vi "Billard2025.vi"(5 "Open PDF":bool=TRUE, 7 "Diamètre balle":i32=13, 8 "ColorchocWin":u32(colorbox), 9 "ColorchocLose":u32(colorbox), 10 "Create scoresheet":bool=TRUE, 11 "Path":path) -> (0 "Error out":errorcluster, 1 "Summary":string)   [LabVIEW 2025]
panel:
  out "?":string="Billard 2025"
  out "BANCKEN Thomas 393134\n\nDELAMARE Romain 373041\n\nDIEBOLD Jules 393356":string="BANCKEN Thomas 393134\n\nDELAMARE Romain 373041\n\nDIEBOLD Jules 393356"
  out "?":string="Auteurs"
  out "PNG Picture":picture
  out "Output cluster":errorcluster
  in  "LineStyle":enum16{"-", "--", ":", "-."}(ring)=enum."--"
  in  "MarkerStyle":enum16{"o", "+", "*", ".", "x", "s", "d"}(ring)=enum."*"
  # "(Doit etre compris entre 10 & 15)"
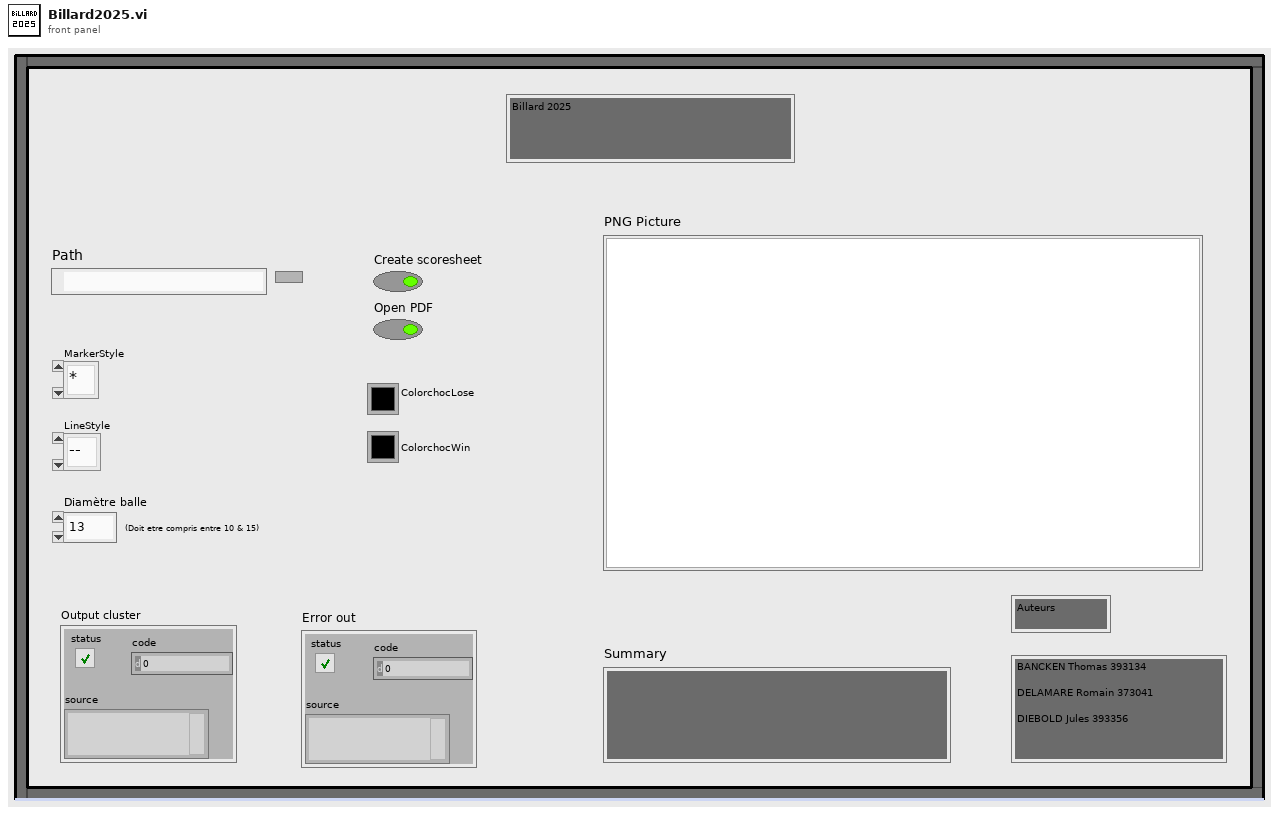
[diagram p1: front panel]
types:
  T1 = cluster{"Bottom":dbl, "Top":dbl, "Left":dbl, "Right":dbl}
  T2 = cluster{"Xr":i32, "Yr":i32, "Sr":i32, "Xy":i32, "Yy":i32, "Sy":i32, "Xw":i32, "Yw":i32, "Sw":i32}
  T3 = enum16{"open", "replace", "create", "open or create", "replace or create", "replace or create with confirmation"}
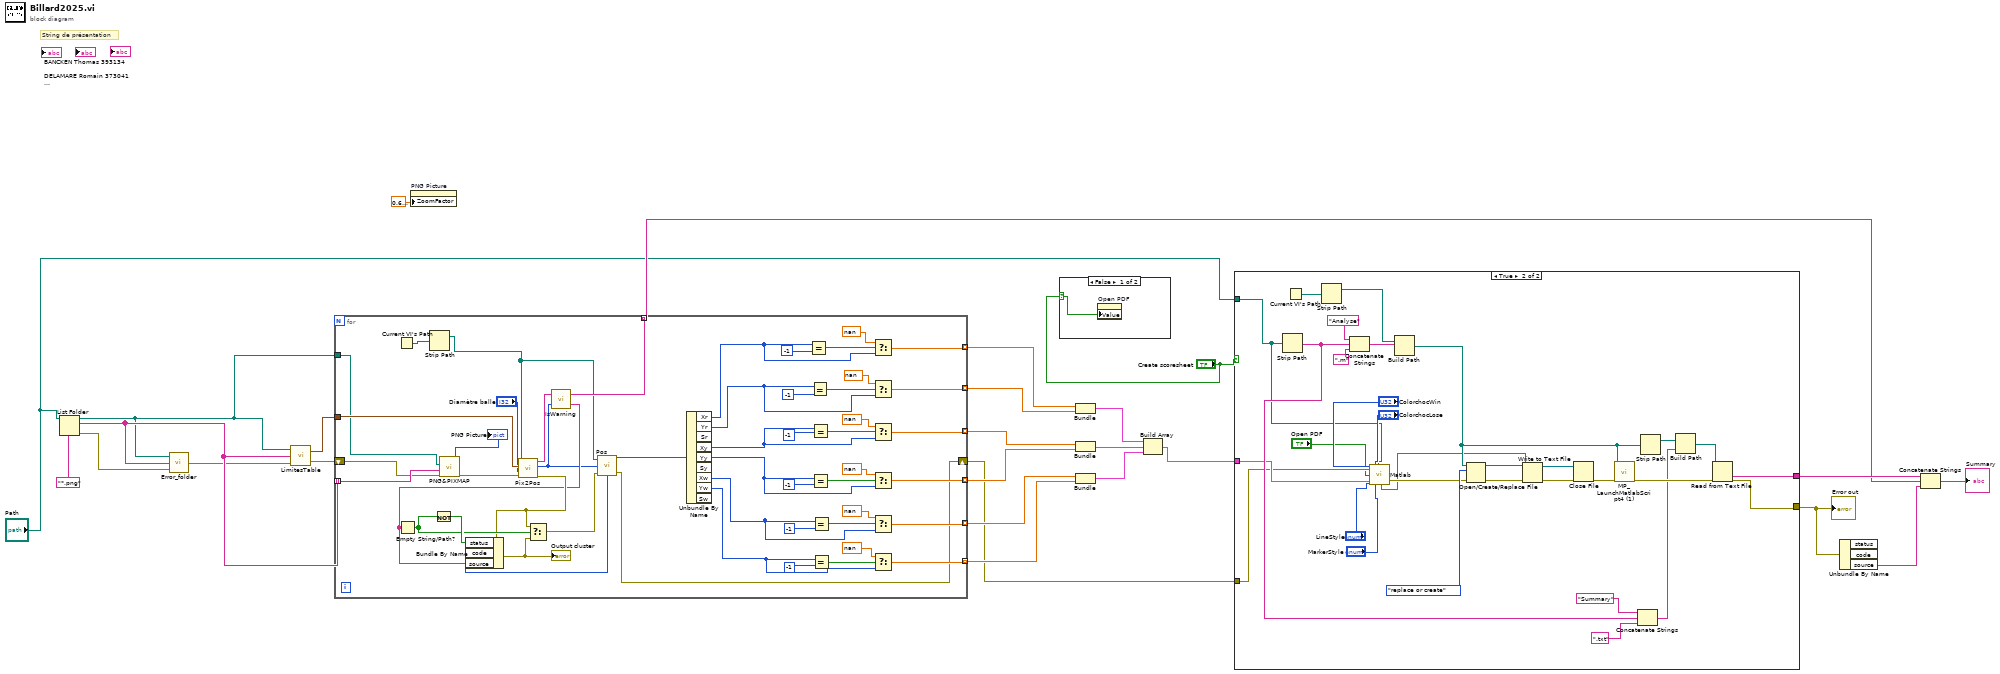
[diagram p0: block diagram]
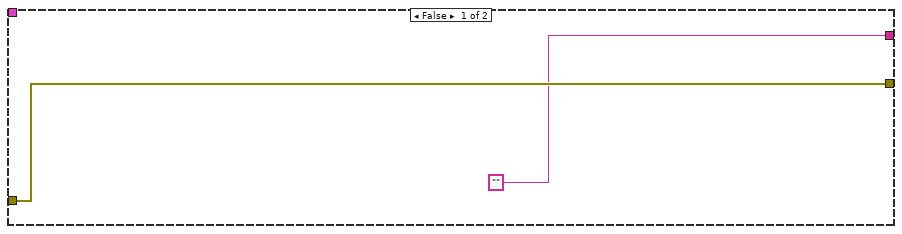
[diagram p3: hidden frame]
diagram:
  # "String de présentation"
  n1 = List Folder(path="Path", pattern="*.png") -> (path out=w4:path, filenames=w12:string[], error out=w11:errorcluster)  [unwired: 2 in, 1 out]
  n2 = call "Error_folder.vi"("error in"=w11, "File PNG"=w12, "Folder Path"=w4) -> ("error out"=w2:errorcluster)
  n3 = call "LimitesTable.vi"("error in"=w2, "PNGs in folder"=w12, "Folder path"=w4) -> ("error out"=w14:errorcluster, "Billard rect"=w26:T1)
  n4 = for {
    tunnel: w26 -> [w76]
    tunnel: w12 -> [w75] mode=indexing
    tunnel: [w49] -> w24 mode=indexing
    tunnel: [w48] -> w20 mode=indexing
    tunnel: [w47] -> w19 mode=indexing
    tunnel: [w46] -> w18 mode=indexing
    tunnel: [w45] -> w23 mode=indexing
    tunnel: [w44] -> w17 mode=indexing
    shift-right: [w38] -> w3
    shift-left: w14 -> [w43]
    tunnel: [w30] -> w6 mode=indexing
    tunnel: w4 -> [w28]
    n5 = Current VI's Path() -> (path=w29:path)
    n6 = Strip Path(path=w29) -> (stripped path=w27:path)  [unwired: 1 out]
    n7 = call "PNG&PIXMAP.vi"("error in"=w43, "Current png filename"=w75, "Png path"=w28) -> ("error out"=w42:errorcluster, "PNG Picture"=→"PNG Picture":picture)  [unwired: 4 in, 1 out]
    n8 = call "Pix2Pos.vi"("error in"=w42, "Diamètre balle"="Diamètre balle", "Billard rect"=w76, "path fichier"=w27) -> ("error out"=w36:errorcluster, "Return code C"=w33:i32, "Stderr du C"=w34:string)  [unwired: 5 in]
    n9 = call "IsWarning.vi"("Numeric"=w33, "error string in"=w34) -> ("Error string out"=w35:string, "Warning"=w30:string)
    n10 = Empty String/Path?(string/path=w35) -> (empty?=w40:bool)
    n11 = Not(x=w40) -> (.not. x?=w41:bool)
    n12 = Bundle By Name(cluster=w36, "status"=w41, "code"=w33, "source"=w35) -> (w32:errorcluster)
    "Output cluster" <- w32
    n13 = Select(t=w36, s=w40, f=w32) -> (s? t:f=w31:errorcluster)
    n14 = call "Pos.vi"("error in"=w31, "name or relative path"=w27) -> ("error out"=w38:errorcluster, "output cluster"=w74:T2)  [unwired: 2 in]
    n15 = Unbundle By Name(w74) -> ("Xr"=w55:i32, "Yr"=w54:i32, "Xy"=w53:i32, "Yy"=w52:i32, "Xw"=w51:i32, "Yw"=w50:i32)  [unwired: 3 out]
    n16 = Equal?(x=w55, y=-1) -> (x = y?=w67:bool)
    n17 = Equal?(x=w54, y=-1) -> (x = y?=w66:bool)
    n18 = Equal?(x=w53, y=-1) -> (x = y?=w65:bool)
    n19 = Equal?(x=w52, y=-1) -> (x = y?=w64:bool)
    n20 = Equal?(x=w51, y=-1) -> (x = y?=w63:bool)
    n21 = Equal?(x=w50, y=-1) -> (x = y?=w62:bool)
    n22 = Select(t=nan, s=w67, f=w55) -> (s? t:f=w49:dbl)
    n23 = Select(t=nan, s=w66, f=w54) -> (s? t:f=w48:dbl)
    n24 = Select(t=nan, s=w65, f=w53) -> (s? t:f=w47:dbl)
    n25 = Select(t=nan, s=w64, f=w52) -> (s? t:f=w46:dbl)
    n26 = Select(t=nan, s=w63, f=w51) -> (s? t:f=w45:dbl)
    n27 = Select(t=nan, s=w62, f=w50) -> (s? t:f=w44:dbl)
  }
  n28 = property on="PNG Picture" class="Pict"("ZoomFactor"=sgl 0.7 ("Zoom Factor")) -> ()  [unwired: 2 in, 2 out]
  n29 = case shown="False" "Create scoresheet" {
    selector: "Create scoresheet" -> [w77 _]
    frame False {
      n30 = property on="Open PDF" class="Bool (strict)"("Value"=w77) -> ()  [unwired: 2 in, 2 out]
    }
    frame True {
    }
  }
  n31 = Bundle(w24, w20) -> (w22:cluster{dbl[], dbl[]})  [unwired: 1 in]
  n32 = Bundle(w19, w18) -> (w16:cluster{dbl[], dbl[]})  [unwired: 1 in]
  n33 = Bundle(w23, w17) -> (w15:cluster{dbl[], dbl[]})  [unwired: 1 in]
  n34 = Build Array(w22, w16, w15) -> (w21:cluster{dbl[], dbl[]}[])
  n35 = case shown="True" "Create scoresheet" {
    tunnel: w21 -> [_ w88]
    tunnel: "Path" -> [_ w82]
    tunnel: w3 -> [w79 w87]
    tunnel: [w79 w94] -> w7
    tunnel: ["" w103] -> w10
    frame False {
    }
    frame True {
      n36 = Strip Path(path=w82) -> (name=w96:string)  [unwired: 1 out]
      n37 = Current VI's Path() -> (path=w81:path)
      n38 = Strip Path(path=w81) -> (stripped path=w80:path)  [unwired: 1 out]
      n39 = Concatenate Strings("Analyse", w96, ".m") -> (w108:string)
      n40 = call "Matlab.vi"("ColorchocWin"="ColorchocWin", "error in"=w87, "Boolean"="Open PDF", "Ball Coordinates"=w88, "LineStyle"="LineStyle", "ColorchocLoose"="ColorchocLose", "MarkerStyle"="MarkerStyle", "Path"=w82) -> ("Script"=w84:string, "error out"=w91:errorcluster)  [unwired: 10 in]
      n41 = Build Path(base path=w80, name or relative path=w108) -> (appended path=w93:path)
      n42 = Open/Create/Replace File(file path (use dialog)=w93, error in=w91, operation (0:open)=T3."replace or create") -> (refnum out=w107:refnum<file>, error out=w106:errorcluster)  [unwired: 3 in, 1 out]
      n43 = Write to Text File(file (use dialog)=w107, text=w84, error in=w106) -> (refnum out=w97:refnum<file>, error out=w105:errorcluster)  [unwired: 1 in, 1 out]
      n44 = Close File(refnum=w97, error in=w105) -> (error out=w104:errorcluster)  [unwired: 1 out]
      n45 = call "MP_LaunchMatlabScript4 (1).vi"("error in (no error)"=w104, "matlab script path"=w93) -> ("error out"=w102:errorcluster)  [unwired: 4 in, 5 out]
      n46 = Concatenate Strings("Summary", w96, ".txt") -> (w99:string)
      n47 = Strip Path(path=w93) -> (stripped path=w92:path)  [unwired: 1 out]
      n48 = Build Path(base path=w92, name or relative path=w99) -> (appended path=w98:path)
      n49 = Read from Text File(file (use dialog)=w98, error in=w102) -> (text=w103:string, error out=w94:errorcluster)  [unwired: 2 in, 2 out]
    }
  }
  "Error out" <- w7
  n50 = Unbundle By Name(w7) -> ("source"=w8:string)  [unwired: 2 out]
  n51 = Concatenate Strings(w10, w6, w8) -> (→"Summary":string)
